vi "Timing Engine.vi"(8 "error in":errorcluster, 9 "Time Limit":dbl, 10 "Reset":bool, 11 "Advance Time?":bool) -> (0 "error out":errorcluster, 1 "Elapsed Time":dbl, 3 "Time Expired?":bool)   [LabVIEW 2016]
doc: "This VI will take the timestamp each time it is called determine \"dt\" - change in time between calls. If the \"Advance Time?\" input is true, dt will be added to the elapsed time which is stored in this VI. The elapsed time will be reset to 0 if the \"Reset\" Input is True. The \"Time Limit\" input will be compared to the elapsed time to determine if the time has expired."
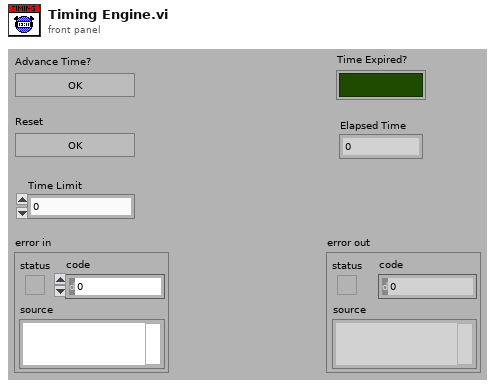
[diagram p1: front panel]
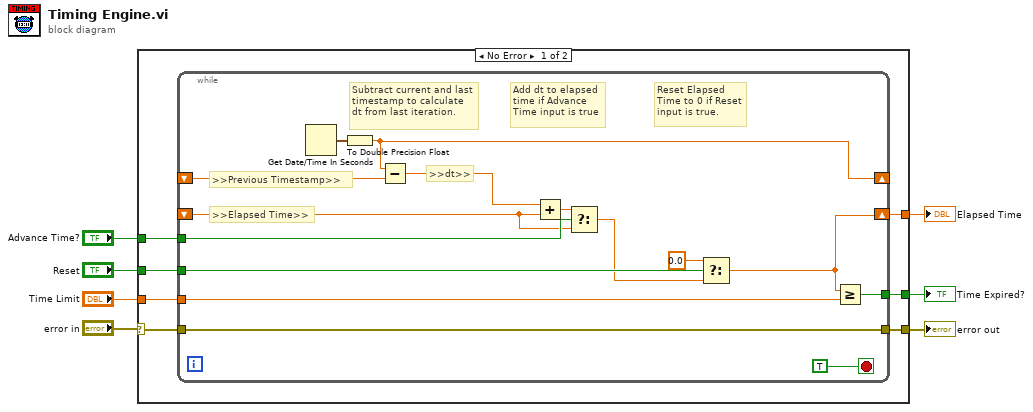
[diagram p0: block diagram]
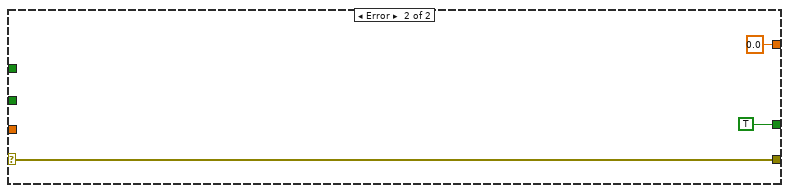
[diagram p2: hidden frame]
diagram:
  n1 = case shown="No Error" "error in" {
    selector: "error in" -> [w8 w32]
    tunnel: "Reset" -> [w14 _]
    tunnel: [w13 0.0 ("t")] -> w6
    tunnel: "Time Limit" -> [w12 _]
    tunnel: [w11 TRUE] -> w4
    tunnel: "Advance Time?" -> [w10 _]
    tunnel: [w9 w32] -> w1
    frame No Error {
      n2 = while {
        shift-right: [w27] -> _
        shift-left: _ -> [w26]
        shift-right: [w22] -> w13
        shift-left: _ -> [w17]
        tunnel: w14 -> [w24]
        tunnel: w12 -> [w21]
        tunnel: [w20] -> w11
        tunnel: w10 -> [w19]
        tunnel: [w15] -> w9
        tunnel: w8 -> [w15]
        stop <- TRUE stop-if-true
        # "Reset Elapsed Time to 0 if Reset input is true."
        # "Subtract current and last timestamp to calculate dt from last iteration."
        # "Add dt to elapsed time if Advance Time input is true"
        # ">>dt>>"
        # ">>Elapsed Time>>"
        # ">>Previous Timestamp>>"
        n3 = Get Date/Time In Seconds() -> (seconds since 1Jan1904=w28:timestamp)
        n4 = To Double Precision Float(number=w28) -> (double precision float=w27:dbl)
        n5 = Subtract(x=w27, y=w26) -> (x-y=w25:dbl)
        n6 = Add(x=w25, y=w17) -> (x+y=w18:dbl)
        n7 = Select(t=w18, s=w19, f=w17) -> (s? t:f=w16:dbl)
        n8 = Select(t=0.0, s=w24, f=w16) -> (s? t:f=w22:dbl)
        n9 = Greater Or Equal?(x=w22, y=w21) -> (x >= y?=w20:bool)
      }
    }
    frame Error {
    }
  }
  "Elapsed Time" <- w6
  "Time Expired?" <- w4
  "error out" <- w1
